vi "SUB_SearchFile_inFolderAdvance.vi"(1 "Find this String":string) -> (0 "File Existing True/Flase":bool)   [LabVIEW 2011]
panel:
  out "String":string
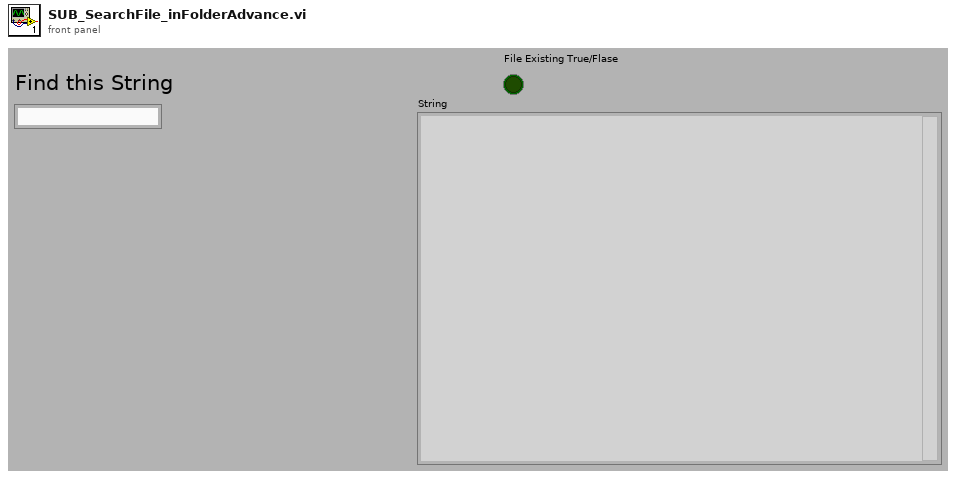
[diagram p1: front panel]
types:
  T1 = enum32{"invalid app kind", "Development System", "Run Time System", "Student Edition", "Embedded LabVIEW", "Evaluation", "Custom"}
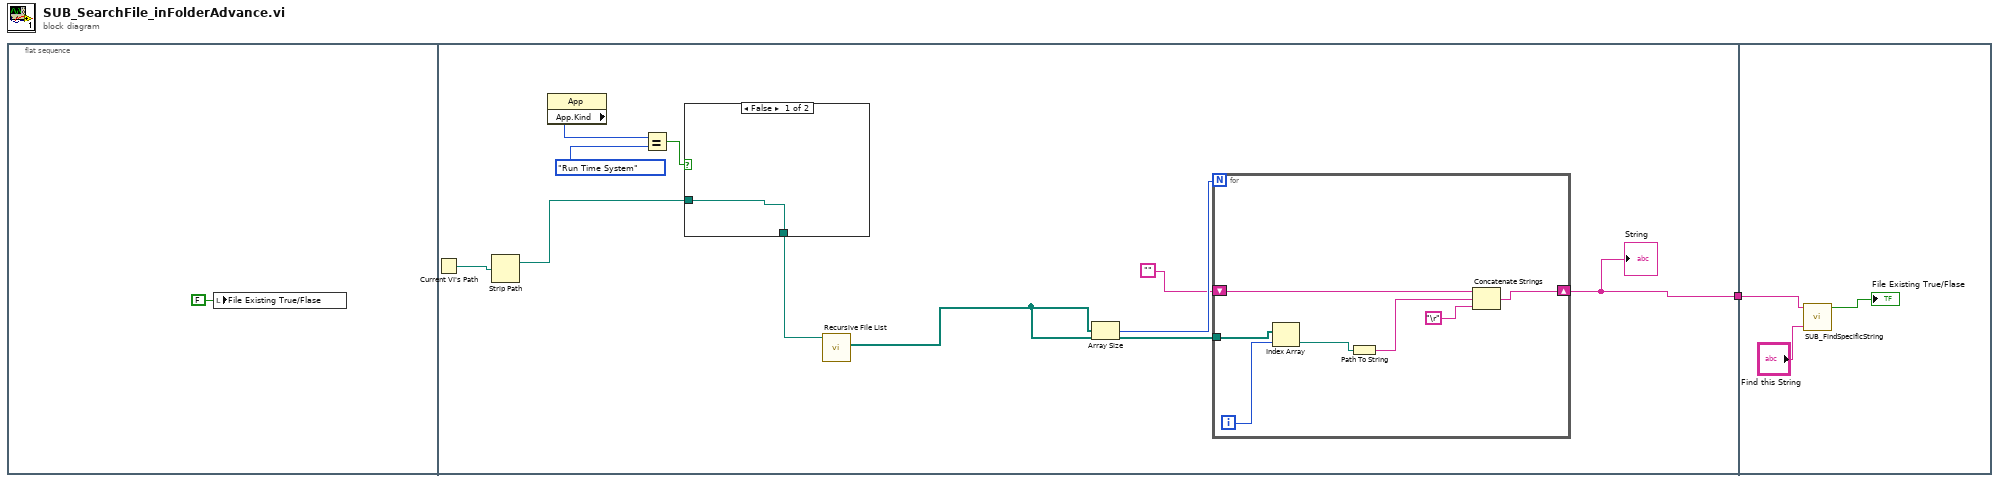
[diagram p0: block diagram]
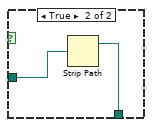
[diagram p2: hidden frame]
diagram:
  n1 = flat-sequence {
    tunnel: [w3] -> w1
    tunnel: w1 -> [w25]
    frame #0 {
      n2 = local write "File Existing True/Flase"(FALSE ("File Existing True/Flase")) -> ()
    }
    frame #1 {
      n3 = Current VI's Path() -> (path=w12:path)
      n4 = Strip Path(path=w12) -> (stripped path=w8:path)  [unwired: 1 out]
      n5 = property class="App"() -> ("App.Kind"=w9:T1)  [unwired: 2 in, 2 out]
      n6 = Equal?(x=w9, y=T1."Run Time System" ("Application:Kind")) -> (x = y?=w11:bool)
      n7 = case shown="False" w11 {
        tunnel: [w20 w22] -> w7
        tunnel: w8 -> [w20 w21]
        frame False {
        }
        frame True {
          n8 = Strip Path(path=w21) -> (stripped path=w22:path)  [unwired: 1 out]
        }
      }
      n9 = call <vilib>:"Recursive File List.vi"("Folder Path"=w7) -> ("All Files in Dir"=w5:path[])  [unwired: 6 in, 4 out]
      n10 = Array Size(array=w5) -> (size(s)=w6:i32)
      n11 = for {
        N: w6 -> [_]
        tunnel: w5 -> [w18]
        shift-right: [w15] -> w3
        shift-left: "" -> [w14]
        i -> [w19]
        n12 = Index Array(array=w18, index=w19) -> (element=w17:path)
        n13 = Path To String(path=w17) -> (string=w16:string)
        n14 = Concatenate Strings(w14, w16, "\r") -> (w15:string)
      }
      "String" <- w3
    }
    frame #2 {
      n15 = call "SUB_FindSpecificString.vi"("Find this String"="Find this String", "String data"=w25) -> ("Found"=→"File Existing True/Flase":bool)  [unwired: 2 in, 1 out]
    }
  }
